vi "GL_Brk_Pt_PRF.vi"(0 "Motion Settings In":T1={"No Motion?"=FALSE, "Motion System"=enum."NI 735x", "Motion Bd ID"=1, "Motion Profile"="SMAC1", "# Axis"=1, "Reverse Z axis?"=TRUE, "SMAC Axis"=0, "scan pair"=enum."y-(x) scan", "RT fps"=6.0, "Steps per mm"=[1000, 1000, 1000, 1000], "Motor Parameters"={"velocity ct/s"=[10000.0, 10000.0, 10000.0, 50000.0], "accel ct/s^2"=[50000.0, 50000.0, 50000.0, 200000.0]}, "One Way Scan"=FALSE, "Reverse One Way Scan"=FALSE, "Global Position (mm)"=[], "Plane"=0, "Distance between\nscan lines (um)"=0.0, "Distance between\nscan planes (um)"=0.0, "number of scan planes"=1, "Total steps in line"=0, "Xtra plane\ndistance  (um)"=100, "Xtra planes "=1, "Add Axis"=FALSE, "overshoot cts"=200, "BKPT Shift"=0, "Scan Start Time (ms)"=0, "ESP VISA"="GPIB::1::INSTR", "3rd Axis"=1, "GL Ref Out"=refnum, "Galil Address"=""} {"3rd Axis" items=["x", "y", "z", "w"]; "Xtra planes" min=1; "Xtra plane\ndistance  (um)" min=0; "Distance between\nscan planes (um)" format="%.2f"; "Distance between\nscan lines (um)" format="%.2f"; "SMAC Axis" items=["None"=0, "Axis 1"=1, "Axis 2"=2, "Axis 3"=3, "Axis 4"=4, "Axis 5"=5, "Axis 6"=6, "Axis 7"=7, "Axis 8"=8, "Vector Space 1"=17, "Vector Space 2"=18, "Vector Space 3"=19, "Vector Space 4"=20]; "Motion Bd ID" min=1 max=32 step=1}, 1 "Axis":u16(ring)=1 items=["Axis 1"=1, "Axis 2"=2, "Axis 3"=3, "Axis 4"=4, "Axis 5"=5, "Axis 6"=6, "Axis 7"=7, "Axis 8"=8], 2 "Reverse ?":bool, 11 "error in (no error)":errorcluster, 13 "Offset":i32) -> (3 "ref out":refnum<k7>, 4 "Start Position":i32, 6 "End Position":i32, 10 "Motion error":bool, 15 "error out":errorcluster)   [LabVIEW 2022 SP3]
doc: "EXAMPLE: DO_WHILE Loop (Onboard Programming Template)\n\nSUMMARY:\nThis FlexMotion example demonstrates the implementation of a DO_WHILE loop data structure in an onboard program. The C equivalent of the data structure implemented here is:\n\ndo {\n// code to be repeated\nloopVar = loopVar - increment;\n} while (loopVar != 0);\n\nTHEORY OF OPERATION:\nThe flow of the DO_WHILE loop data structure goes as follows:\n(1) Program storage is begun.\n(2) The DO_WHILE loop is set up. (Loop Variable and Increment are each defined and initialized.)\n(3) A code delimiter is set using label #1.\n(4) Code to be executed each time through loop is run (in the template program, the loop variable is decremented).\n(5) The loop variable or other test condition is checked.\n(6) If the test condition is true, then we jump back to label #1. Otherwise, the condition is false so the loop terminates.\n(7) Program storage is ended.\n\nDEVELOPMENT DETAILS:\nApplication Software: LabVIEW 5.0.x\nHardware: FlexMotion controller\nDriver Software: FlexMotion Software 4.0\n\nREQUIRED HARDWARE:\n(controller only)\n\nINSTRUCTIONS:\n(0) Initialize the FlexMotion controller before running this VI. \n(1) Add the FlexMotion functions you want to execute into the block diagram where noted.\n(2) Run the VI to store the program. (The program will not be executed at this time.)\n(3) You can then run the program you have stored by calling the run_prog.flx function with the appropriate program number.\n\nADDITIONAL NOTES:\n(a) You should read the following items before writing FlexMotion onboard programs:\n(1) The Onboard Programs section of the FlexMotion Hardware User Manual (page 4-9 in the November 1998 edition).\n(2) The section about onboard variables in your FlexMotion Software Reference Manual (pages 4-11 and 4-12 in the November 1998 edition)\n(3) You will find the chapter of the FlexMotion Software Reference Manual concerning the Onboard Programming functions to be an invaluable reference resource (Chapter 12 of the November 1998 edition) along with the online help for the VI functions.\n(b) This template repeats the DO_WHILE loop as long as an expression with a variable evaluates to be true. However, you may evaluate other conditions such as move complete status instead.\n\n*NOTE: This example is not supported on the 7334 controller."
uses:
  NI_controller/-NI_MotionRoutines/MotionParameters.ctl
  NI_controller/-NI_MotionRoutines/MotionSys.ctl
  -MotionRoutines/ScanAxis.ctl
  -MotionRoutines/3rdAxis.ctl
  Command Menu.ctl
  -MotionRoutines/MotionGlobals.vi
  Pulsers/PulserGlobals.vi
  <instrlib>/Newport ESP301/Newport ESP301.lvlib
panel:
  out "Motion stop loop":i32
  # "Doesn't seem to work. Too much overhead to maintain PRF"
  # "1-D and 2-D B scan settings"
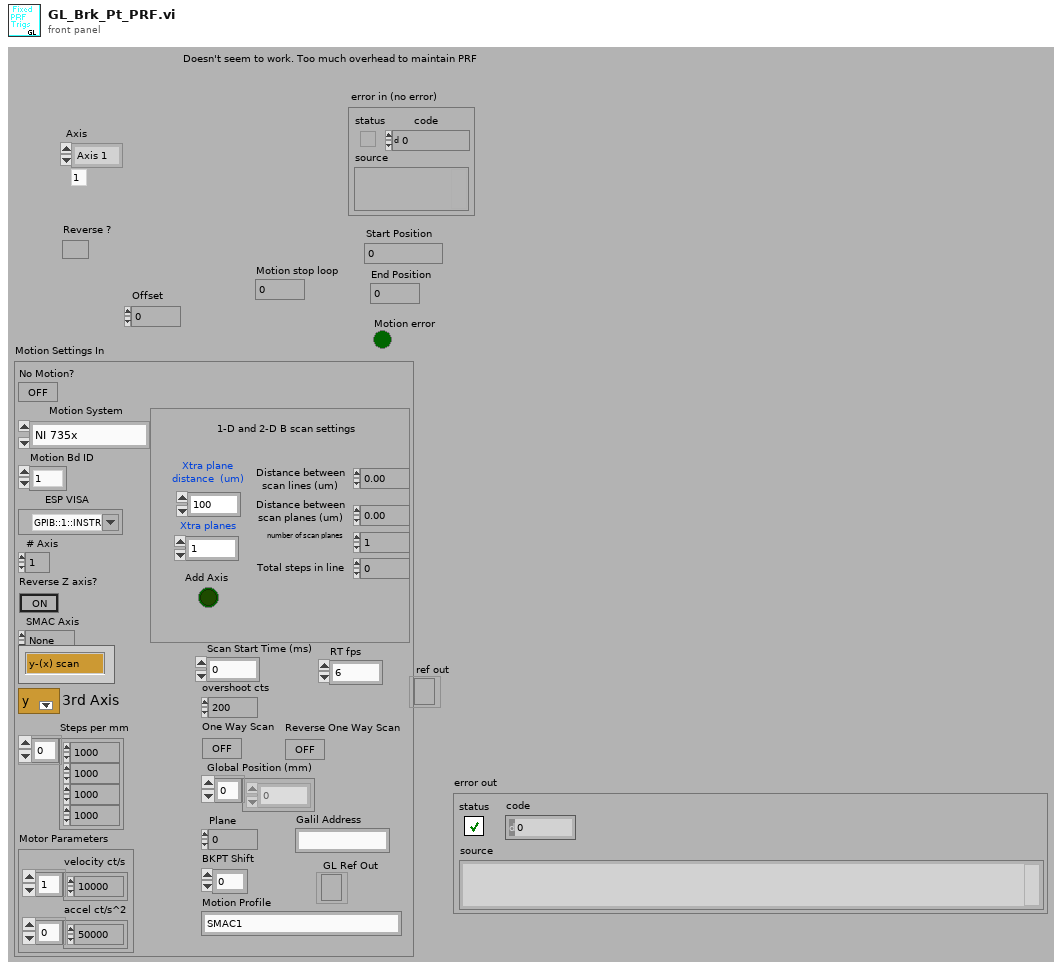
[diagram p1: front panel]
types:
  T1 = typedef "MotionParameters.ctl" = cluster{"No Motion?":bool, "Motion System":T2, "Motion Bd ID":u8, "Motion Profile":string, "# Axis":i8, "Reverse Z axis?":bool, "SMAC Axis":u16, "scan pair":T3, "RT fps":sgl, "Steps per mm":i32[], "Motor Parameters":cluster{"velocity ct/s":dbl[], "accel ct/s^2":dbl[]}, "One Way Scan":bool, "Reverse One Way Scan":bool, "Global Position (mm)":dbl[], "Plane":i32, "Distance between\nscan lines (um)":sgl, "Distance between\nscan planes (um)":sgl, "number of scan planes":i32, "Total steps in line":i32, "Xtra plane\ndistance  (um)":i32, "Xtra planes ":i32, "Add Axis":bool, "overshoot cts":i32, "BKPT Shift":i32, "Scan Start Time (ms)":u32, "ESP VISA":refnum<visa-resource-name>, "3rd Axis":T4, "GL Ref Out":refnum<k7>, "Galil Address":string}
  T2 = typedef "MotionSys.ctl" = enum16{"MM3000", "NI 735x", "Newport ESP", "No Motion Card", "Galil"}
  T3 = typedef "ScanAxis.ctl" = enum16{"y-(x) scan", "x-(y) scan", "z-(x) scan", "z-(y) scan", "y-(z) scan", "x-(z) scan", "w-(x) scan", "w-(y) scan", "w-(z) scan", "x-(w) scan", "y-(w) scan", "z-(w) scan"}
  T4 = typedef "3rdAxis.ctl" = u16
  T5 = typedef "Command Menu.ctl" = enum16{"CommandPassThrough", "Abort Motion", "Define Pos", "Velocity", "Acceleration", "Deceleration", "Position Rel", "Postion Abs", "Begin Move", "After Move", "Home", "KI", "KD", "KP", "IL", "Config I/O", "Set Bit", "Clear Bit", "Motor Off", "Moto On", "Status", "Execute", "Halt Execute", "HX Status", "Tell Velocity", "Check Motion", "BreakPoint", "Tell Position", "Current Code Line", "Tell Switches", "OC Force On", "OC Off", "Pos Soft Limit", "Rev Soft Limit"}
  T6 = enum16{"Absolute Position", "Relative Position", "Velocity", "Relative to Cap Pos", "Modulus Position", "Absolute Contouring", "Relative Contouring"}
  T7 = typedef "GL Axis Control.ctl" = u16
  T8 = enum16{"Less Than", "Equal", "Less Than Or Equal", "Greater Than", "Not Equal", "Greater Than Or Equal", "True", "Home Found", "Index Found", "High Speed Capture", "Position Breakpoint", "Reserved", "Velocity Threshold", "Move Complete", "Profile Complete", "Blend Complete", "Motor Off", "Home Input Active", "Limit Input Active", "Software Limit Active", "Program Complete", "IO Port Match"}
  T9 = typedef "location.ctl" = enum16{"Automatic", "WCM Main", "Hawaii", "Columbia MM3000", "Columbia  NI System", "NYU", "RRI 2", "UHI Allen", "CUMC RT", "Chiba", "Stony Brook", "WCM Microscopy", "WCM Aeoretch", "WCM Optics Lab", "WCM Main 2Axis", "WCM Rotation", "WCM SAM SMAC", "SERI GP"}
  T10 = cluster{"Port A bit-0 at logic level":bool, "Port A bit-1 at logic level":bool, "Port A bit-2 at logic level ":bool, "Port A bit-3 at logic level":bool, "Port A bit-4 at logic level":bool, "Port A bit-5 at logic level ":bool, "Port A bit-6 at logic level ":bool, "Port A bit-7 at logic level ":bool, "Port B bit-0 at logic level":bool, "Port B bit-1 at logic level":bool, "Port B bit-2 at logic level ":bool, "Port B bit-3 at logic level":bool, "Port B bit-4 at logic level":bool, "Port B bit-5 at logic level ":bool, "Port B bit-6 at logic level ":bool, "Port B bit-7 at logic level ":bool}
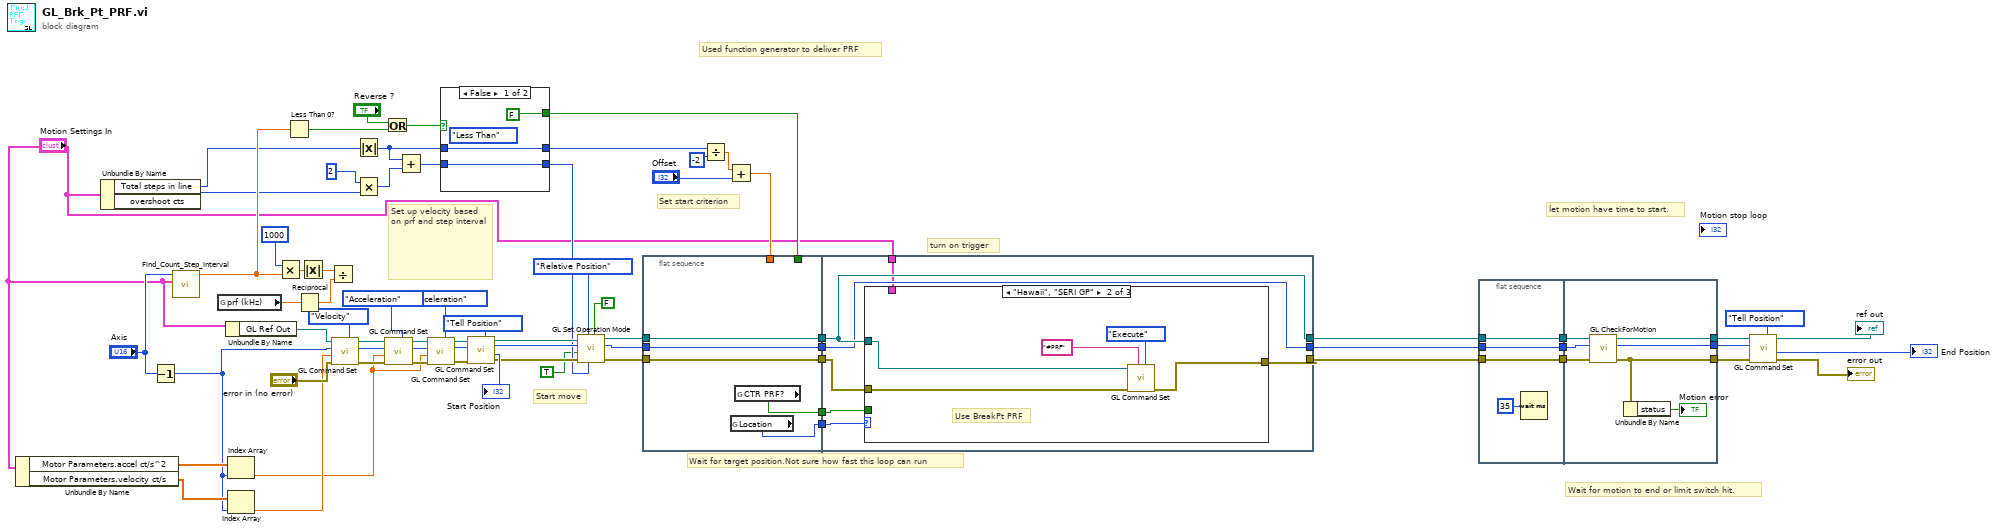
[diagram p0: block diagram]
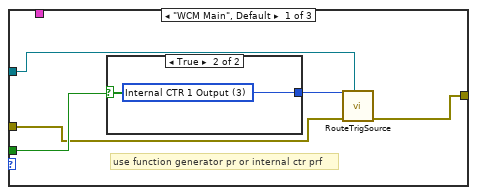
[diagram p2: hidden frame]
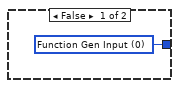
[diagram p3: hidden frame]
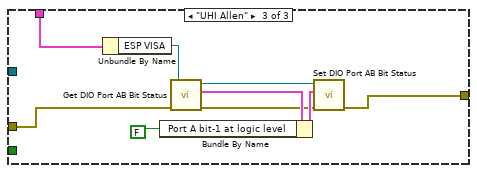
[diagram p4: hidden frame]
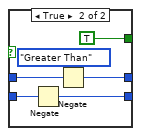
[diagram p5: hidden frame]
diagram:
  # "Wait for motion to end or limit switch hit."
  # "let motion have time to start."
  # "Used function generator to deliver PRF"
  # "turn on trigger"
  # "Wait for target position.Not sure how fast this loop can run"
  # "Set start criterion"
  # "Set up velocity based on prf and step interval"
  # "Start move"
  n1 = Unbundle By Name("Motion Settings In") -> ("Motor Parameters.accel ct/s^2"=w49:dbl[], "Motor Parameters.velocity ct/s"=w48:dbl[])
  n2 = Unbundle By Name("Motion Settings In") -> ("Total steps in line"=w44:i32, "overshoot cts"=w45:i32)
  n3 = Decrement(x="Axis") -> (x-1=w33:u16)
  n4 = call "Find_Count_Step_Interval.vi"("Motion Settings In"="Motion Settings In", "Axis"="Axis") -> ("BP Interval"=w46:dbl)  [unwired: 8 in, 1 out]
  n5 = global read "PulserGlobals.vi" "prf (kHz)"() -> (w43:dbl)
  n6 = Unbundle By Name("Motion Settings In") -> ("GL Ref Out"=w40:refnum<k7>)
  n7 = Index Array(array=w49, index=w33) -> (element=w31:dbl)
  n8 = Index Array(array=w48, index=w33) -> (element=w32:dbl)
  n9 = Multiply(x=1000, y=w46) -> (x*y=w54:dbl)
  n10 = Less Than 0?(x=w46) -> (x < 0?=w72:bool)
  n11 = Reciprocal(x=w43) -> (1/x=w61:dbl)
  n12 = Absolute Value(x=w54) -> (abs(x)=w68:dbl)
  n13 = Divide(x=w68, y=w61) -> ()  [unwired: 1 out]
  n14 = call "GL Command Set.vi"("Command"=Command_Menu."Velocity", "error in (no error)"="error in (no error)", "Value"=w32, "Axis"=w33, "Galil.IGalil"=w40) -> ("error out"=w41:errorcluster, "Axis Out"=w38:T7, "ref out"=w42:refnum<k7>)  [unwired: 2 in, 2 out]
  n15 = Absolute Value(x=w44) -> (abs(x)=w67:i32)
  n16 = Multiply(x=2, y=w45) -> (x*y=w52:i32)
  n17 = Or(x="Reverse ?", y=w72) -> (x .or. y?=w70:bool)
  n18 = call "GL Command Set.vi"("Command"=Command_Menu."Acceleration", "error in (no error)"=w41, "Value"=w31, "Axis"=w38, "Galil.IGalil"=w42) -> ("error out"=w36:errorcluster, "Axis Out"=w35:T7, "ref out"=w37:refnum<k7>)  [unwired: 2 in, 2 out]
  n19 = Add(x=w67, y=w52) -> (x+y=w69:i32)
  n20 = call "GL Command Set.vi"("Command"=Command_Menu."Deceleration", "error in (no error)"=w36, "Value"=w31, "Axis"=w35, "Galil.IGalil"=w37) -> ("error out"=w27:errorcluster, "Axis Out"=w25:T7, "ref out"=w28:refnum<k7>)  [unwired: 2 in, 2 out]
  n21 = case shown="False" w70 {
    tunnel: w69 -> [w75 w80]
    tunnel: [w75 w79] -> w19
    tunnel: [w74 w77] -> w63
    tunnel: w67 -> [w74 w78]
    tunnel: [FALSE TRUE] -> w59
    frame False {
      (unwired) T8."Less Than" ("Condition Code (True)")
    }
    frame True {
      (unwired) T8."Greater Than" ("Condition Code (True)")
      n22 = Negate(x=w80) -> (-x=w79:i32)
      n23 = Negate(x=w78) -> (-x=w77:i32)
    }
  }
  n24 = call "GL Command Set.vi"("Command"=Command_Menu."Tell Position", "error in (no error)"=w27, "Axis"=w25, "Galil.IGalil"=w28) -> ("error out"=w22:errorcluster, "Response#"=→"Start Position":i32, "Axis Out"=w21:T7, "ref out"=w23:refnum<k7>)  [unwired: 3 in, 1 out]
  n25 = call "GL Set Operation Mode.vi"("LimitWarning?"=FALSE, "position cts (abs/rel)"=w19, "Position Mode (Absolute)"=T6."Relative Position", "error in (no error)"=w22, "Start Now?"=TRUE, "Axis"=w21, "Galil.IGalil"=w23) -> ("error out"=w16:errorcluster, "Axis Out Output"=w12:T7, "Galil Out"=w17:refnum<k7>)  [unwired: 2 in]
  n26 = flat-sequence {
    tunnel: w60 -> [_]
    tunnel: w59 -> [_]
    tunnel: [w84] -> w57
    tunnel: [w85] -> w56
    tunnel: w17 -> [w84]
    tunnel: w16 -> [w85]
    tunnel: [w83] -> w13
    tunnel: w12 -> [w83]
    tunnel: [w82] -> w3
    tunnel: [w81] -> w2
    tunnel: [w92] -> w58
    tunnel: [w88] -> w62
    tunnel: w57 -> [w88]
    tunnel: w56 -> [w91]
    tunnel: [w87] -> w15
    tunnel: w13 -> [w87]
    tunnel: w3 -> [w90]
    tunnel: w2 -> [w89]
    tunnel: "Motion Settings In" -> [w86]
    frame #0 {
      n27 = global read "MotionGlobals.vi" "Location"() -> (w81:T9)
      n28 = global read "MotionGlobals.vi" "CTR PRF?"() -> (w82:bool)
    }
    frame #1 {
      n29 = case shown="\"Hawaii\", \"SERI GP\"" w89 {
        tunnel: w90 -> [w97 _ _]
        tunnel: [w95 w102 w107] -> w92
        tunnel: w91 -> [w94 w101 w108]
        tunnel: w88 -> [w93 w100 _]
        tunnel: w86 -> [_ _ w106]
        frame "WCM Main", Default {
          # "use function generator pr or internal ctr prf"
          n30 = case shown="True" w97 {
            tunnel: [w98 w99] -> w96
            frame False {
              w98 = u16 0 items=["Function Gen Input", "Motion Trig", "Internal RT Motion Trig", "Internal CTR 1 Output"] ("Trig Source")
            }
            frame True {
              w99 = u16 3 items=["Function Gen Input", "Motion Trig", "Internal RT Motion Trig", "Internal CTR 1 Output"] ("Trig Source")
            }
          }
          n31 = call "RouteTrigSource.vi"("Galil.IGalil"=w93, "error in"=w94, "Trig Source"=w96) -> ("error out"=w95:errorcluster)  [unwired: 8 in]
        }
        frame "Hawaii", "SERI GP" {
          # "Use BreakPt PRF"
          n32 = call "GL Command Set.vi"("Command"=Command_Menu."Execute", "Text Input"="#PRF", "error in (no error)"=w101, "Galil.IGalil"=w100) -> ("error out"=w102:errorcluster)  [unwired: 3 in, 4 out]
        }
        frame "UHI Allen" {
          n33 = Unbundle By Name(w106) -> ("ESP VISA"=w105:refnum<visa-resource-name>)
          n34 = call <instrlib>:"Get DIO Port AB Bit Status.vi"("error in (no error)"=w108, "VISA resource name"=w105) -> ("error out"=w110:errorcluster, "DIO Port A status"=w113:T10, "VISA resource name out"=w109:refnum<visa-resource-name>)  [unwired: 3 in]
          n35 = Bundle By Name(cluster=w113, "Port A bit-1 at logic level"=FALSE) -> (w111:T10)
          n36 = call <instrlib>:"Set DIO Port AB Bit Status.vi"("error in (no error)"=w110, "DIO Port status"=w111, "VISA resource name"=w109) -> ("error out"=w107:errorcluster)  [unwired: 3 in, 1 out]
        }
      }
    }
  }
  n37 = Divide(x=w63, y=-2) -> (x/y=w65:dbl)
  n38 = Add(x=w65, y="Offset") -> (x+y=w60:dbl)
  n39 = flat-sequence {
    tunnel: w62 -> [w116]
    tunnel: [w116] -> w51
    tunnel: w58 -> [w115]
    tunnel: [w115] -> w50
    tunnel: w15 -> [w114]
    tunnel: [w114] -> w14
    tunnel: w51 -> [w123]
    tunnel: w50 -> [w122]
    tunnel: [w121] -> w9
    tunnel: [w120] -> w8
    tunnel: w14 -> [w119]
    tunnel: [w118] -> w10
    frame #0 {
      n40 = Wait (ms)(milliseconds to wait=35) -> ()  [unwired: 1 out]
    }
    frame #1 {
      n41 = call "GL CheckForMotion.vi"("error in"=w122, "Axis"=w119, "Refnum in"=w123) -> ("error out"=w120:errorcluster, "Axis out"=w118:T7, "Refnum out"=w121:refnum<k7>)  [unwired: 6 in]
      n42 = Unbundle By Name(w120) -> ("status"=→"Motion error":bool)
    }
  }
  n43 = call "GL Command Set.vi"("Command"=Command_Menu."Tell Position", "error in (no error)"=w8, "Axis"=w10, "Galil.IGalil"=w9) -> ("error out"=→"error out":errorcluster, "Response#"=→"End Position":i32, "ref out"=→"ref out":refnum<k7>)  [unwired: 3 in, 2 out]
